vi "Stop Core.vi"(10 "final error code":i32 caption="最终错误代码", 11 "LS-H600-TCP Client in":refnum<class "LS-H600-TCP Client.lvclass"> caption="操作者输入") -> (3 "LS-H600-TCP Client out":refnum<class "LS-H600-TCP Client.lvclass"> caption="操作者输出")   [LabVIEW 2022 SP3, in "LS-H600-TCP Client.lvlib" / "LS-H600-TCP Client.lvclass"]
doc: "(<B>Filename</B>: Actor Framework.lvlib:Actor.lvclass:Stop Core.vi)\n\nDefines what the actor does before it stops. Use the <B>final error code</B> input to determine whether the actor shut down in response to an error.\n\nBy default, this method does nothing.子孙类重写该方法，定义出错时的操作，例如，关闭操作者核心方法初始的进程。"
uses:
  LS-H600-TCP Client.lvclass
  <vilib>/ActorFramework/Actor/Actor.lvclass
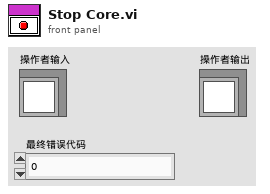
[diagram p1: front panel]
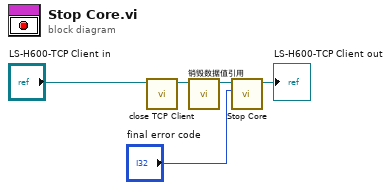
[diagram p0: block diagram]
diagram:
  n1 = call "close TCP Client.vi"("LS-H600-TCP Client 输入"="LS-H600-TCP Client in") -> ("LS-H600-TCP Client 输出"=w3:refnum<class "LS-H600-TCP Client.lvclass">)  [unwired: 9 in, 1 out]
  n2 = call "销毁数据值引用.vi"("LS-H600-TCP Client 输入"=w3) -> ("LS-H600-TCP Client 输出"=w2:refnum<class "LS-H600-TCP Client.lvclass">)  [unwired: 9 in, 1 out]
  n3 = call-parent "Stop Core.vi"("final error code"="final error code", "Actor in"=w2) -> ("Actor out"=→"LS-H600-TCP Client out":refnum<class "LS-H600-TCP Client.lvclass">)  [unwired: 9 in]
